vi "Initialize Device Core.vi"(8 "error in (no error)":errorcluster, 9 "Reset (F)":bool, 10 "Resource Name":string, 11 "IVI_DMM_Delayed in":refnum<class "IVI_DMM_Delayed.lvclass">) -> (0 "error out":errorcluster, 3 "IVI_DMM_Delayed out":refnum<class "IVI_DMM_Delayed.lvclass">)   [LabVIEW 2015, in "IVI_DMM.lvlib" / "IVI_DMM_Delayed.lvclass"]
doc: "Initialize device driver."
uses:
  IVI_DMM_Delayed.lvclass
  IVI_DMM_Delayed.lvclass/IVI_DMM_Delayed.ctl
  IVI_DMM/IVI_DMM.lvclass
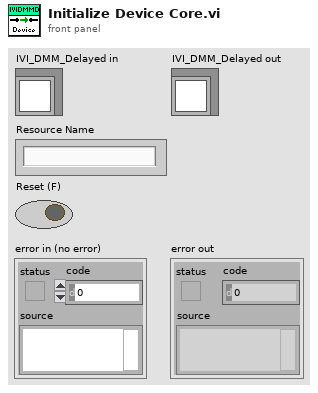
[diagram p1: front panel]
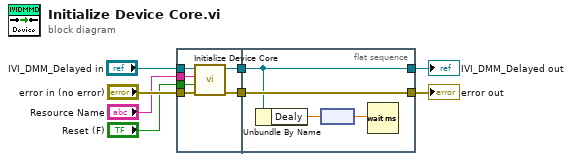
[diagram p0: block diagram]
diagram:
  n1 = flat-sequence {
    tunnel: "error in (no error)" -> [w12]
    tunnel: "Reset (F)" -> [w11]
    tunnel: "Resource Name" -> [w10]
    tunnel: "IVI_DMM_Delayed in" -> [w9]
    tunnel: [w14] -> w2
    tunnel: [w13] -> w1
    tunnel: [w15] -> w7
    tunnel: [w18] -> w8
    tunnel: w2 -> [w18]
    tunnel: w1 -> [w15]
    frame #0 {
      n2 = call-parent "Initialize Device Core.vi"("error in (no error)"=w12, "Reset (F)"=w11, "Resource Name"=w10, "IVI_DMM in"=w9) -> ("error out"=w14:errorcluster, "IVI_DMM out"=w13:refnum<class "IVI_DMM_Delayed.lvclass">)  [unwired: 6 in]
    }
    frame #1 {
      n3 = Unbundle By Name(w15) -> ("Dealy"=w16:dbl[unit])
      n4 = node(w16) -> (w17:dbl)
      n5 = Wait (ms)(milliseconds to wait=w17) -> ()  [unwired: 1 out]
    }
  }
  "error out" <- w8
  "IVI_DMM_Delayed out" <- w7
